vi "Undistort.vi"   [LabVIEW 2020, in "ar.lvlib"]
doc: "Undistorts the Source image to correct for the Distortion values on the Camera Parameters.\n\nIf more control over the undistortion process is required or if the same Distortion needs to be corrected in multiple images then use the \"Image Undistorter.lvclass\" to avoid duplicate calculations."
uses:
  ar.lvlib
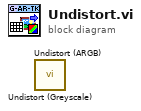
[diagram p0: block diagram]
diagram:
  n1 = call "Undistort (Greyscale).vi"() -> ()  [unwired: 10 in, 2 out]
  n2 = call "Undistort (ARGB).vi"() -> ()  [unwired: 10 in, 2 out]
